vi "Toolbar Manage Button Click Event.vi"(6 "Index In":i32, 8 "error in (no Error)":errorcluster, 9 "Button Index":i32, 10 "Button States In":refnum<class "Button.lvclass">[](array[class]), 11 "Data In":T1) -> (0 "error out":errorcluster, 1 "Data Changed ?":bool, 2 "Button States Out":refnum<class "Button.lvclass">[](array[class]), 3 "Data Out":T1, 4 "Index Out":i32)   [LabVIEW 2012, in "Toolbar.xctl"]
doc: "Process Left Button Clicks on the toolbar taking account of the button state and type."
uses:
  Toolbar.xctl
  Button_Class/Button.lvclass
  Toolbar Data.ctl
  Button_Class/Type Defs/Button Events.ctl
  Button_Class/Type Defs/Button Status.ctl
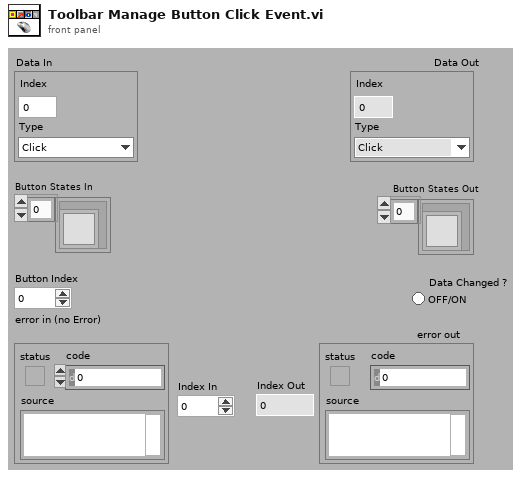
[diagram p1: front panel]
types:
  T1 = typedef "Toolbar.xctl/Toolbar Data.ctl" = cluster{"Index":i32, "Type":T2}
  T2 = typedef "Button.lvclass/Button Events.ctl" = enum16{"Click", "Latch", "Unlatch"}
  T3 = typedef "Button.lvclass/Button Status.ctl" = enum16{"Off", "Hover", "On", "Disabled"}
  T4 = typedef "Button.lvclass/Button Type.ctl" = enum16{"Transitory", "Latching"}
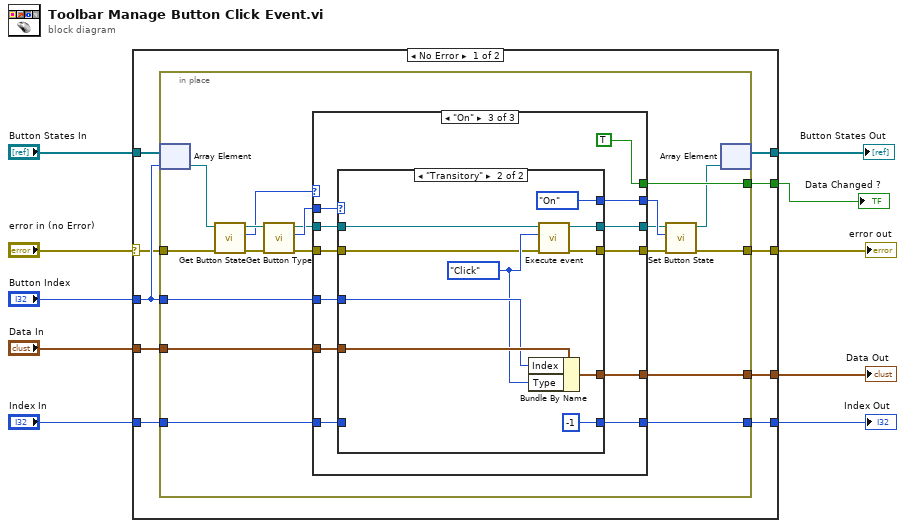
[diagram p0: block diagram]
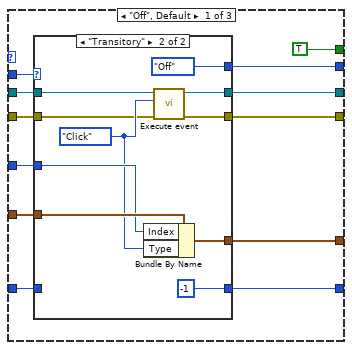
[diagram p2: hidden frame]
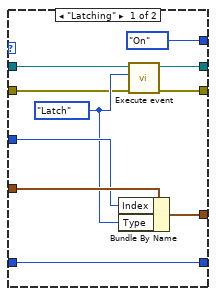
[diagram p3: hidden frame]
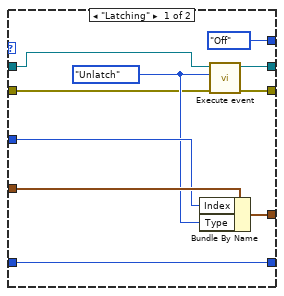
[diagram p5: hidden frame]
diagram:
  n1 = case shown="No Error" "error in (no Error)" {
    selector: "error in (no Error)" -> [w15 w111]
    tunnel: [w20 _] -> w10
    tunnel: [w19 _] -> w9
    tunnel: "Button Index" -> [w18 _]
    tunnel: "Button States In" -> [w17 _]
    tunnel: [w16 w110] -> w6
    tunnel: [w14 w111] -> w4
    tunnel: "Data In" -> [w13 w110]
    tunnel: [w12 w109] -> w2
    tunnel: "Index In" -> [w11 w109]
    frame No Error {
      n2 = in-place {
        in-place-border: w18 -> [w23]
        in-place-border: w13 -> [w39]
        in-place-border: [w38] -> w14
        in-place-border: w15 -> [w37]
        in-place-border: [w36] -> w20
        in-place-border: [w35] -> w16
        in-place-border: [w22] -> w12
        in-place-border: w11 -> [w21]
        n3 = in-place-array #1(w17, w18) -> (w25:refnum<class "Button.lvclass">)
        n4 = call-dynamic "Get Button State.vi"("error in (no error)"=w37, "Button in"=w25) -> ("error out"=w28:errorcluster, "State"=w32:T3, "Button out"=w33:refnum<class "Button.lvclass">)  [unwired: 7 out]
        n5 = call-dynamic "Get Button Type.vi"("error in (no error)"=w28, "Button in"=w33) -> ("error out"=w26:errorcluster, "Type"=w31:T4, "Button out"=w30:refnum<class "Button.lvclass">)  [unwired: 7 out]
        n6 = case shown="\"On\"" w32 {
          selector: w32 -> [_ w76 _]
          tunnel: [w42 w76 w79] -> w34
          tunnel: [w50 w75 w86] -> w35
          tunnel: w39 -> [w49 w75 w88]
          tunnel: w23 -> [w47 _ w87]
          tunnel: [TRUE _ TRUE] -> w36
          tunnel: w31 -> [w48 _ w85]
          tunnel: w30 -> [w46 w74 w84]
          tunnel: [w45 w74 w83] -> w29
          tunnel: [w43 w73 w82] -> w27
          tunnel: w26 -> [w44 w73 w81]
          tunnel: [w40 w72 w77] -> w22
          tunnel: w21 -> [w41 w72 w78]
          frame "Off", Default {
            n7 = case shown="\"Transitory\"" w48 {
              tunnel: w49 -> [w61 w71]
              tunnel: [w60 w70] -> w50
              tunnel: w47 -> [w59 w69]
              tunnel: w46 -> [w58 w68]
              tunnel: [w57 w67] -> w45
              tunnel: w44 -> [w55 w65]
              tunnel: [w54 w64] -> w43
              tunnel: [Button_Status."On" ("t") Button_Status."Off" ("t")] -> w42
              tunnel: [w52 -1 ("Index In")] -> w40
              tunnel: w41 -> [w52 _]
              frame "Latching" {
                w56 = Button_Events."Latch" ("Type")
                n8 = Bundle By Name(cluster=w61, "Index"=w59, "Type"=w56) -> (w60:T1)
                n9 = call-dynamic "Execute event.vi"("error in (no error)"=w55, "Button Event"=w56, "Button in"=w58) -> ("error out"=w54:errorcluster, "Button out"=w57:refnum<class "Button.lvclass">)  [unwired: 1 in, 6 out]
              }
              frame "Transitory" {
                w66 = Button_Events."Click" ("Type")
                n10 = Bundle By Name(cluster=w71, "Index"=w69, "Type"=w66) -> (w70:T1)
                n11 = call-dynamic "Execute event.vi"("error in (no error)"=w65, "Button Event"=w66, "Button in"=w68) -> ("error out"=w64:errorcluster, "Button out"=w67:refnum<class "Button.lvclass">)  [unwired: 1 in, 6 out]
              }
            }
          }
          frame "Disabled" {
          }
          frame "On" {
            n12 = case shown="\"Transitory\"" w85 {
              tunnel: w88 -> [w98 w108]
              tunnel: [w97 w107] -> w86
              tunnel: w87 -> [w96 w106]
              tunnel: w84 -> [w95 w105]
              tunnel: [w94 w103] -> w83
              tunnel: w81 -> [w92 w101]
              tunnel: [w91 w102] -> w82
              tunnel: [Button_Status."Off" ("State") Button_Status."On" ("State")] -> w79
              tunnel: [w89 -1 ("Index In")] -> w77
              tunnel: w78 -> [w89 _]
              frame "Latching" {
                w93 = Button_Events."Unlatch" ("Type")
                n13 = Bundle By Name(cluster=w98, "Index"=w96, "Type"=w93) -> (w97:T1)
                n14 = call-dynamic "Execute event.vi"("error in (no error)"=w92, "Button Event"=w93, "Button in"=w95) -> ("error out"=w91:errorcluster, "Button out"=w94:refnum<class "Button.lvclass">)  [unwired: 1 in, 6 out]
              }
              frame "Transitory" {
                w104 = Button_Events."Click" ("Type")
                n15 = Bundle By Name(cluster=w108, "Index"=w106, "Type"=w104) -> (w107:T1)
                n16 = call-dynamic "Execute event.vi"("error in (no error)"=w101, "Button Event"=w104, "Button in"=w105) -> ("error out"=w102:errorcluster, "Button out"=w103:refnum<class "Button.lvclass">)  [unwired: 1 in, 6 out]
              }
            }
          }
        }
        n17 = call-dynamic "Set Button State.vi"("error in (no error)"=w27, "State"=w34, "Button in"=w29) -> ("error out"=w38:errorcluster, "Button out"=w24:refnum<class "Button.lvclass">)  [unwired: 7 out]
        n18 = in-place-array #1(w24) -> (w19:refnum<class "Button.lvclass">[])  [unwired: 1 out]
      }
    }
    frame Error {
    }
  }
  "Data Changed ?" <- w10
  "Button States Out" <- w9
  "Data Out" <- w6
  "error out" <- w4
  "Index Out" <- w2
